vi "Draw Control Image.vi"(7 "Padding (6px)":i32=6, 9 "Image":T1, 10 "Picture Ref":refnum<vi>) -> ()   [LabVIEW 2020, in "VolatusGUIEditor.lvlib"]
uses:
  VolatusGUIEditor.lvlib
  <vilib>/picture/picture.llb/imagedata.ctl
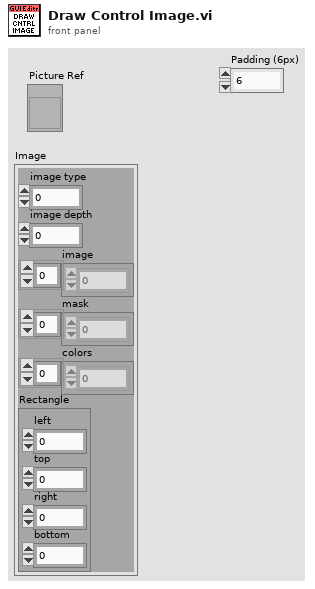
[diagram p1: front panel]
types:
  T1 = typedef "imagedata.ctl" = cluster{"image type":i32, "image depth":i32, "image":u8[], "mask":u8[], "colors":u32[], "Rectangle":cluster{"left":i16, "top":i16, "right":i16, "bottom":i16}}
  T2 = cluster{"left":i16, "top":i16, "right":i16, "bottom":i16}
  T3 = typedef "LVBoundsTypeDef.ctl" = cluster{"Width":u32, "Height":u32}
  T4 = cluster{"left":i32, "top":i32, "right":i32, "bottom":i32}
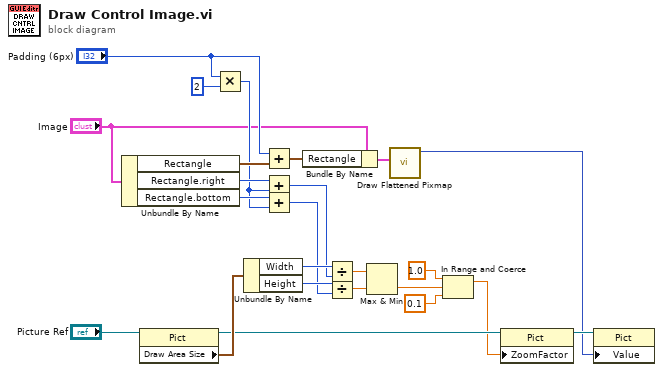
[diagram p0: block diagram]
diagram:
  n1 = Unbundle By Name("Image") -> ("Rectangle"=w15:T2, "Rectangle.right"=w18:i16, "Rectangle.bottom"=w19:i16)
  n2 = property class="Pict"(reference="Picture Ref") -> (reference out=w8:refnum<vi>, "Draw Area Size"=w23:T3)  [unwired: 1 in, 1 out]
  n3 = Multiply(x="Padding (6px)", y=2) -> (x*y=w11:i32)
  n4 = Unbundle By Name(w23) -> ("Width"=w21:u32, "Height"=w20:u32)
  n5 = Add(x="Padding (6px)", y=w15) -> (x+y=w9:T4)
  n6 = Add(x=w18, y=w11) -> (x+y=w12:i32)
  n7 = Add(x=w19, y=w11) -> (x+y=w13:i32)
  n8 = Bundle By Name(cluster="Image", "Rectangle"=w9) -> (w2:T1)
  n9 = Divide(x=w21, y=w12) -> (x/y=w17:dbl)
  n10 = Divide(x=w20, y=w13) -> (x/y=w16:dbl)
  n11 = Max & Min(x=w17, y=w16) -> (min(x,y)=w7:dbl)  [unwired: 1 out]
  n12 = call <vilib>:"Draw Flattened Pixmap.vi"("image data"=w2) -> ("new picture"=w1:picture)  [unwired: 8 in]
  n13 = In Range and Coerce(upper limit=1.0, x=w7, lower limit=0.1) -> (coerced(x)=w4:dbl)  [unwired: 1 out]
  n14 = property class="Pict"(reference=w8, "ZoomFactor"=w4) -> (reference out=w3:refnum<vi>)  [unwired: 1 in, 1 out]
  n15 = property class="Pict"(reference=w3, "Value"=w1) -> ()  [unwired: 1 in, 2 out]
